vi "Harv_2_9.vi"(0 "HarvSetpoints":dbl[](array[numeric]), 1 "Fire":bool, 2 "WinchDown":bool, 3 "HarvPivUP":bool, 5 "HarvPot":dbl, 7 "Count":i32, 9 "BallAcquired":bool, 11 "FireBallSen":bool, 12 "Harvest":bool, 13 "inAuton?":bool, 14 "HarvPivPickupLim":bool) -> (4 "HarvPower":dbl, 6 "HarvRoller":dbl, 8 "CountOut":i32, 10 "HarvStart":bool, 15 "HarvCleared":bool)   [LabVIEW 2013]
panel:
  in  "f":dbl
  in  "MotorScale":dbl=1.5
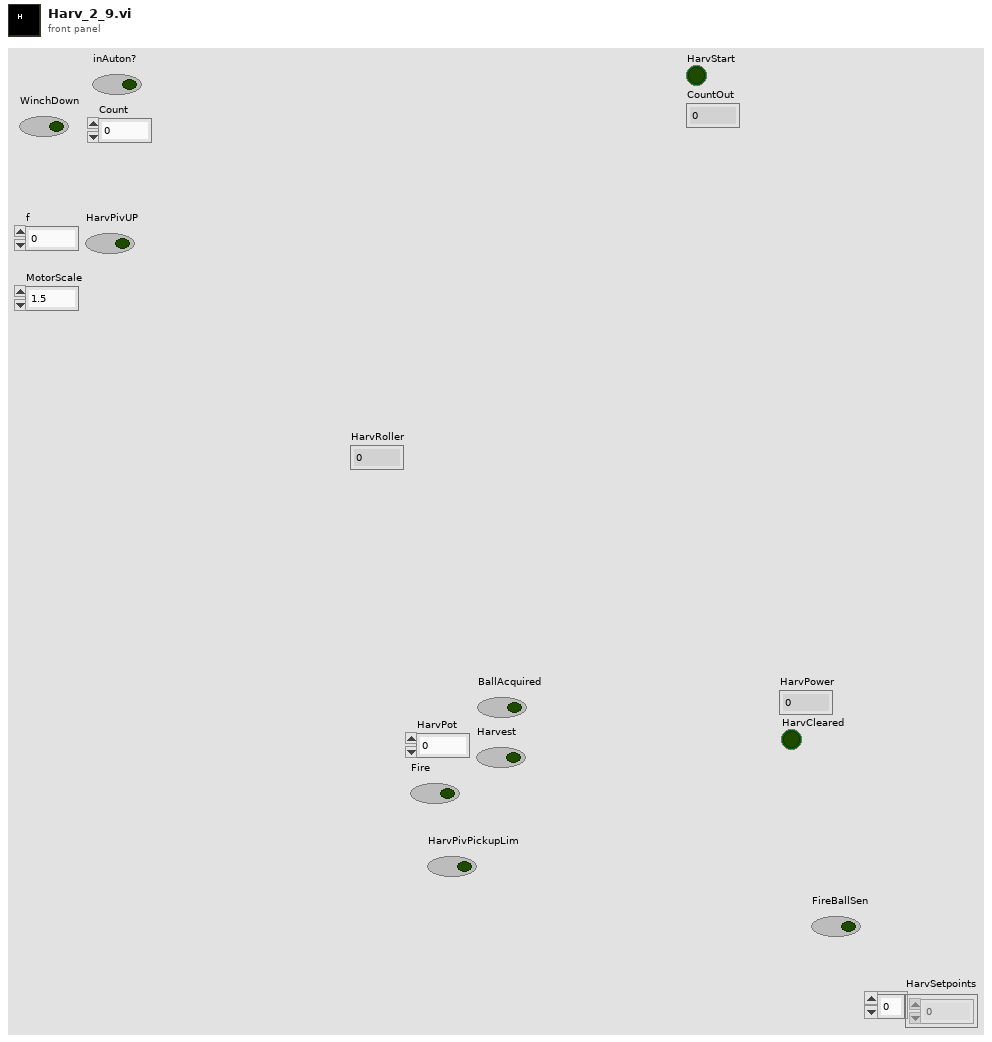
[diagram p1: front panel]
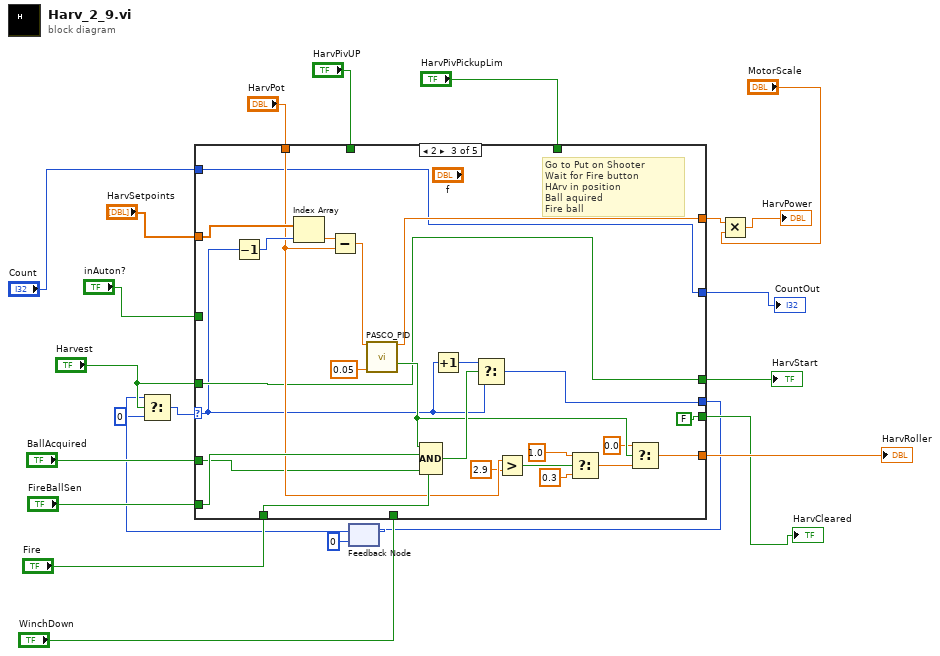
[diagram p0: block diagram]
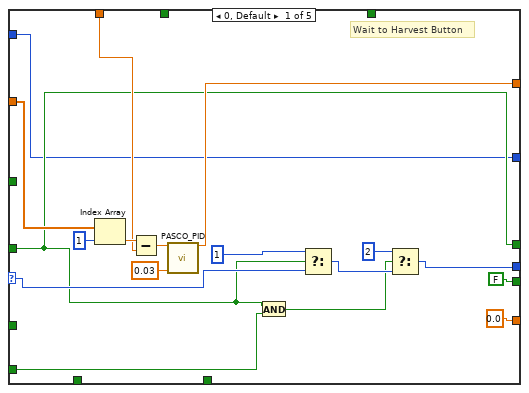
[diagram p2: hidden frame]
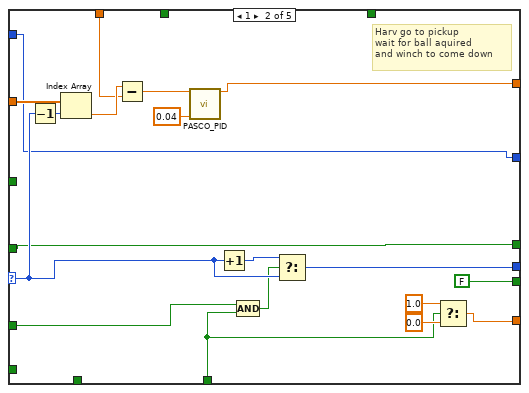
[diagram p3: hidden frame]
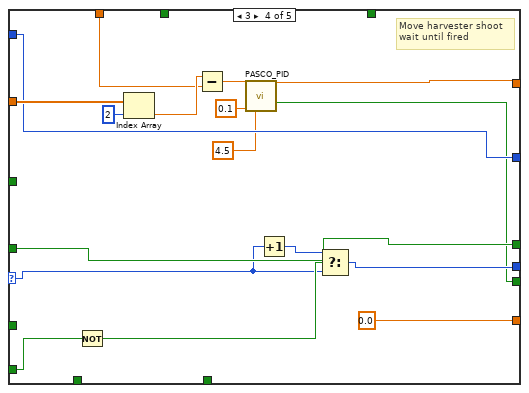
[diagram p4: hidden frame]
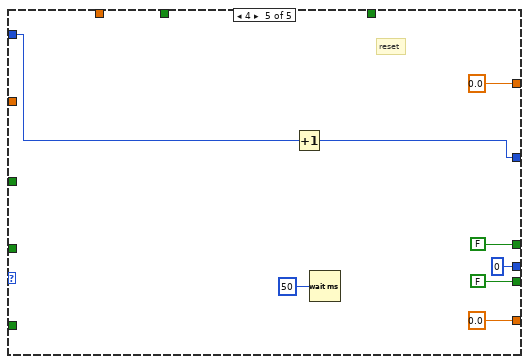
[diagram p5: hidden frame]
diagram:
  n1 = feedback #1(0 ("f")) -> (w15:i32)
  n2 = Select(t=w15, s="Harvest", f=0) -> (s? t:f=w17:i32)
  n3 = case shown="2" w17 {
    selector: w17 -> [w38 w53 w62 w94 _]
    tunnel: "HarvSetpoints" -> [w37 w60 w85 w101 _]
    tunnel: "HarvPot" -> [w36 w58 w76 w91 _]
    tunnel: [w31 w43 w64 w89 0.0 ("Output")] -> w14
    tunnel: [w26 w55 w82 w99 0 ("t")] -> w4
    tunnel: [0.0 ("f") w47 w69 0.0 ("f") 0.0 ("f")] -> w21
    tunnel: "BallAcquired" -> [_ w49 w65 _ _]
    tunnel: "FireBallSen" -> [w28 _ w80 w97 _]
    tunnel: "Fire" -> [_ _ w79 _ _]
    tunnel: "Harvest" -> [w29 w50 w66 w98 _]
    tunnel: [FALSE ("IsThere") FALSE ("IsThere") FALSE ("IsThere") w88 FALSE ("IsThere")] -> w11
    tunnel: "HarvPivPickupLim" -> [_ _ _ _ _]
    tunnel: "HarvPivUP" -> [_ _ _ _ _]
    tunnel: [w29 w50 w66 w98 FALSE ("Harvest")] -> w8
    tunnel: "WinchDown" -> [_ w44 _ _ _]
    tunnel: "inAuton?" -> [_ _ _ _ _]
    tunnel: [w24 w42 w61 w93 w104] -> w2
    tunnel: "Count" -> [w24 w42 w61 w93 w103]
    frame 0, Default {
      # "Wait to Harvest Button"
      n4 = Index Array(array=w37, index=1) -> (element=w39:dbl)
      n5 = Subtract(x=w39, y=w36) -> (x-y=w40:dbl)
      n6 = call "PASCO_PID.vi"("Delta"=w40, "Deadband"=0.03) -> ("Output"=w31:dbl)  [unwired: 12 in, 1 out]
      n7 = And(x=w29, y=w28) -> (x .and. y?=w27:bool)
      n8 = Select(t=1, s=w29, f=w38) -> (s? t:f=w30:i32)
      n9 = Select(t=2, s=w27, f=w30) -> (s? t:f=w26:i32)
    }
    frame 1 {
      # "Harv go to pickup\nwait for ball aquired\nand winch to come down"
      n10 = Decrement(x=w53) -> (x-1=w54:i32)
      n11 = Index Array(array=w60, index=w54) -> (element=w59:dbl)
      n12 = Subtract(x=w59, y=w58) -> (x-y=w57:dbl)
      n13 = call "PASCO_PID.vi"("Delta"=w57, "Deadband"=0.04) -> ("Output"=w43:dbl)  [unwired: 12 in, 1 out]
      n14 = Increment(x=w53) -> (x+1=w56:i32)
      n15 = Compound Arithmetic op=AND(w49, w44) -> (w48:bool)
      n16 = Select(t=w56, s=w48, f=w53) -> (s? t:f=w55:i32)
      n17 = Select(t=1.0, s=w44, f=0.0) -> (s? t:f=w47:dbl)
    }
    frame 2 {
      # "Go to Put on Shooter\nWait for Fire button\nHArv in position\nBall aquired \nFire ball"
      n18 = Decrement(x=w62) -> (x-1=w78:i32)
      n19 = Index Array(array=w85, index=w78) -> (element=w84:dbl)
      n20 = Subtract(x=w84, y=w76) -> (x-y=w83:dbl)
      n21 = call "PASCO_PID.vi"("Delta"=w83, "Deadband"=0.05) -> ("Output"=w64:dbl, "IsThere"=w68:bool)  [unwired: 12 in]
      n22 = Compound Arithmetic op=AND(w68, w80, w79, w65) -> (w81:bool)
      n23 = Increment(x=w62) -> (x+1=w63:i32)
      n24 = Select(t=w63, s=w81, f=w62) -> (s? t:f=w82:i32)
      n25 = Greater?(x=w76, y=2.9) -> (0:w74:bool)
      n26 = Select(t=1.0, s=w74, f=0.3) -> (s? t:f=w70:dbl)
      n27 = Select(t=0.0, s=w68, f=w70) -> (s? t:f=w69:dbl)
    }
    frame 3 {
      # "Move harvester shoot\nwait until fired"
      n28 = Not(x=w97) -> (.not. x?=w96:bool)
      n29 = Index Array(array=w101, index=2) -> (element=w92:dbl)
      n30 = Subtract(x=w92, y=w91) -> (x-y=w90:dbl)
      n31 = call "PASCO_PID.vi"("Delta"=w90, "Deadband"=0.1, "P Gain"=4.5) -> ("Output"=w89:dbl, "IsThere"=w88:bool)  [unwired: 11 in]
      n32 = Increment(x=w94) -> (x+1=w95:i32)
      n33 = Select(t=w95, s=w96, f=w94) -> (s? t:f=w99:i32)
    }
    frame 4 {
      # "reset"
      n34 = Increment(x=w103) -> (x+1=w104:i32)
      n35 = Wait (ms)(milliseconds to wait=u32 50) -> ()  [unwired: 1 out]
    }
  }
  "HarvRoller" <- w21
  "HarvCleared" <- w11
  "HarvStart" <- w8
  "CountOut" <- w2
  n36 = feedback-in #1(w4) -> ()
  n37 = Multiply(x=w14, y="MotorScale") -> (x*y=→"HarvPower":dbl)
